vi "configure.vi"(7 "Save Data":bool=TRUE, 8 "error in (no error)":errorcluster, 11 "QuadraturePositionDecoder in":refnum<class "QuadraturePositionDecoder.lvclass">) -> (0 "error out":errorcluster, 3 "QuadraturePositionDecoder out":refnum<class "QuadraturePositionDecoder.lvclass">)   [LabVIEW 2014, in "QuadraturePositionDecoder.lvclass"]
uses:
  QuadraturePositionDecoder.lvclass
  QuadraturePositionDecoder.lvclass/QuadraturePositionDecoder.ctl
  <vilib>/DAQmx/create/channels.llb/DAQmx Create Channel (CI-Position-Angular Encoder).vi
  <resource>/objmgr/daqmx.rc
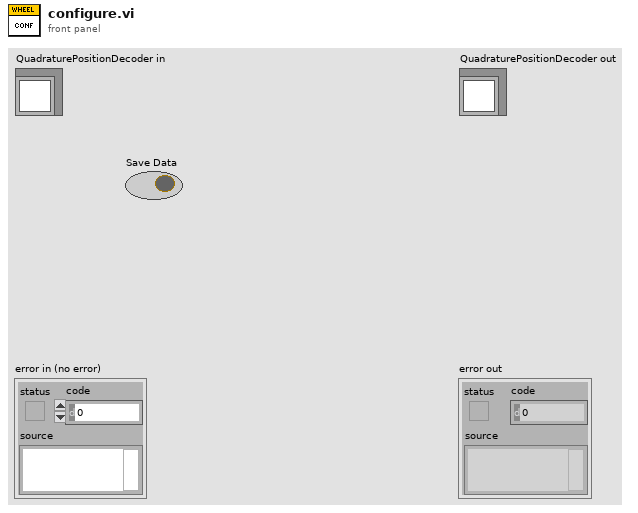
[diagram p1: front panel]
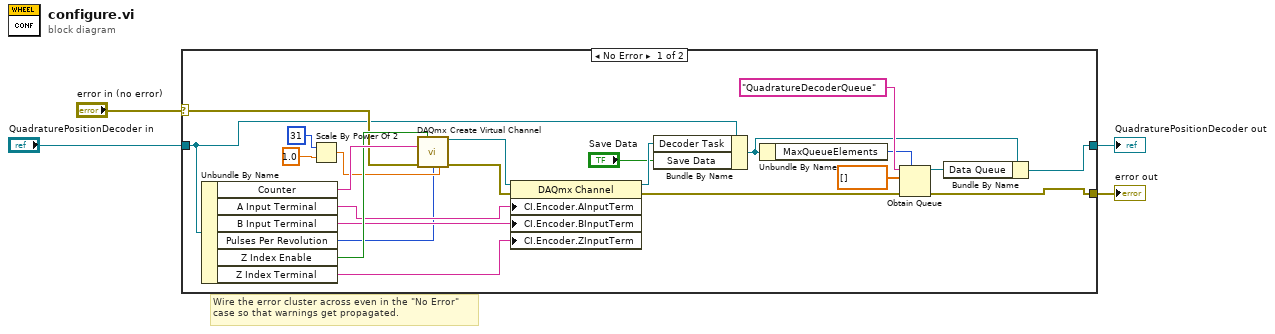
[diagram p0: block diagram]
diagram:
  # "Wire the error cluster across even in the \"No Error\"\ncase so that warnings get propagated."
  n1 = case shown="No Error" "error in (no error)" {
    selector: "error in (no error)" -> [w21 w29]
    tunnel: [w5 w29] -> w3
    tunnel: "QuadraturePositionDecoder in" -> [w7 w28]
    tunnel: [w6 w28] -> w1
    frame No Error {
      n2 = Unbundle By Name(w7) -> ("Counter"=w26:tag, "A Input Terminal"=w24:tag, "B Input Terminal"=w23:tag, "Pulses Per Revolution"=w8:u32, "Z Index Enable"=w25:bool, "Z Index Terminal"=w22:tag)
      n3 = Scale By Power Of 2(n=i16 31, x=1.0) -> (x*2^n=w9:dbl)
      n4 = call-poly <vilib>:"DAQmx Create Virtual Channel.vi"("z index enable"=w25, "counter"=w26, "error in"=w21, "pulses per revolution"=w8, "initial angle"=w9) -> ("task out"=w27:refnum<k21>, "error out"=w20:errorcluster)  [unwired: 9 in]
      n5 = property class="DAQmx Channel"(reference=w27, error in=w20, "CI.Encoder.AInputTerm"=w24, "CI.Encoder.BInputTerm"=w23, "CI.Encoder.ZInputTerm"=w22) -> (reference out=w19:refnum<k21>, error out=w15:errorcluster)
      n6 = Bundle By Name(cluster=w7, "Decoder Task"=w19, "Save Data"="Save Data") -> (w14:refnum<class "QuadraturePositionDecoder.lvclass">)
      n7 = Unbundle By Name(w14) -> ("MaxQueueElements"=w13:i32)
      n8 = Obtain Queue(max queue size (-1, unlimited)=w13, name (unnamed)="QuadratureDecoderQueue", element data type=dbl[] [] ("appended array"), error in (no error)=w15) -> (queue out=w16:refnum<queue>, error out=w5:errorcluster)  [unwired: 1 in, 1 out]
      n9 = Bundle By Name(cluster=w14, "Data Queue"=w16) -> (w6:refnum<class "QuadraturePositionDecoder.lvclass">)
    }
    frame Error {
    }
  }
  "error out" <- w3
  "QuadraturePositionDecoder out" <- w1
